vi "AMB_TCP_Setup.vi"(1 "Host IP":string, 3 "error in (no error)":errorcluster, 4 "Port #":u16) -> (0 "TCP Refnum":u32 format="%.0x", 2 "error out":errorcluster {"code" format="%.0x"})   [LabVIEW 2017]
doc: "Opens and sets up a NI-CAN interface board for use as an AMB master.\nThe CAN Port terminal defaults to CAN0."
panel:
  in  "Numeric":u32
  out "TCP Connection ID":refnum<k5>
  # "ALMA Monitor and Control Bus\nSetup TCP/IP"
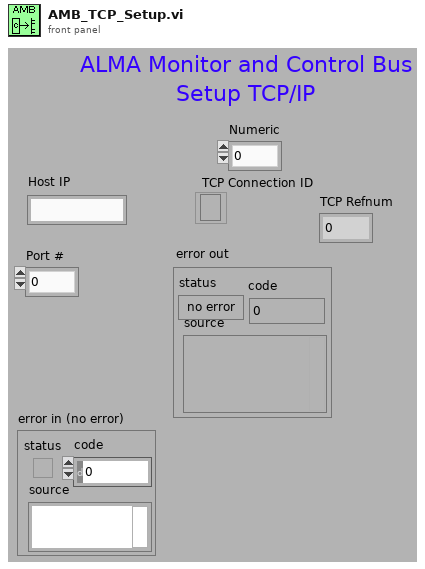
[diagram p1: front panel]
types:
  T1 = cluster{"status":bool, "code":i32, "String To Add":string}
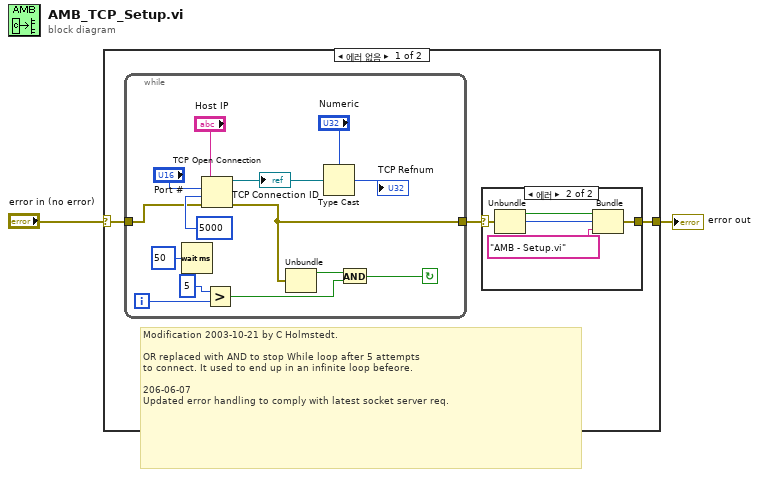
[diagram p0: block diagram]
diagram:
  n1 = case shown="에러 없음" "error in (no error)" {
    selector: "error in (no error)" -> [w5 w26]
    tunnel: [w4 w26] -> w1
    frame No Error {
      # "Modification 2003-10-21 by C Holmstedt.\n\nOR replaced with AND to stop While loop after 5 attempts\nto connect. It used to end up in an infinite loop befeore.\n\n206-06-07\nUpdated error handling to comply with latest socket server req."
      n2 = while {
        tunnel: w5 -> [w13]
        tunnel: [w12] -> w3
        i -> [w17]
        stop <- w18 continue-if-true
        n3 = Wait (ms)(milliseconds to wait=u32 50) -> ()  [unwired: 1 out]
        n4 = TCP Open Connection(address="Host IP", remote port or service name="Port #", timeout ms (60000)=5000, error in (no error)=w13) -> (connection ID=w24:refnum<k5>, error out=w12:errorcluster)  [unwired: 1 in]
        "TCP Connection ID" <- w24
        n5 = Greater?(x=5, y=w17) -> (0:w14:bool)
        n6 = Unbundle(w12) -> ("status"=w20:bool)  [unwired: 2 out]
        n7 = Type Cast(type="Numeric", x=w24) -> (*(type *) &x=→"TCP Refnum":u32)
        n8 = And(x=w20, y=w14) -> (x .and. y?=w18:bool)
      }
      n9 = case shown="에러" w3 {
        selector: w3 -> [w6 w11]
        tunnel: [w6 w8] -> w4
        frame No Error {
        }
        frame Error {
          n10 = Unbundle(w11) -> ("status"=w10:bool, "code"=w9:i32)  [unwired: 1 out]
          n11 = Bundle("status"=w10, "code"=w9, "String To Add"="AMB - Setup.vi") -> (w8:T1)  [unwired: 1 in]
        }
      }
    }
    frame Error {
    }
  }
  "error out" <- w1
